vi "XIPIN_Interleaver_De-interleaver_8_0.vi"   [LabVIEW 2017]
doc: "The Xilinx Interleaver/De-interleaver module is a high speed, compact design and implements either the Forney Convolutional or Rectangular Block type architecture. For the Convolutional type, the number of branches and branch lengths are parameterizable. For the Rectangular Block type the number of rows and columns is parameterizable or run-time variable. Row and column permutations are also supported. The core supports a symbol size ranging from 1 to 256 bits.\n------------------------------------\n<b>Need License</b> : Yes\n<b>Interface</b> : AXI4-Stream"
uses:
  <vilib>/rvi/XilinxIP/XIPIN_XNode/niFpgaXIPIN.xnode
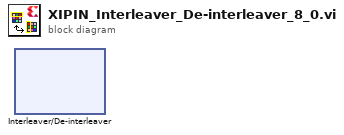
[diagram p0: block diagram]
diagram:
  n1 = xnode ("Interleaver/De-interleaver")() -> ()
